vi "partial derivative.vi"(1 "x":dbl format="%0.2f", 2 "Coefficients":dbl[](array[numeric]) format="%0.2f") -> (0 "Partial Derivative":dbl[](array[numeric]) format="%0.5f")   [LabVIEW 2017, in "NI_AALPro.lvlib"]
uses:
  NI_AALPro.lvlib
panel:
  # "Partial Derivative"
  # "This VI takes an input x along with a number of coefficients to use in the Target Func NonLin vi and does a numerical computation of the partial derivative of the function with repect to each coefficient at value x."
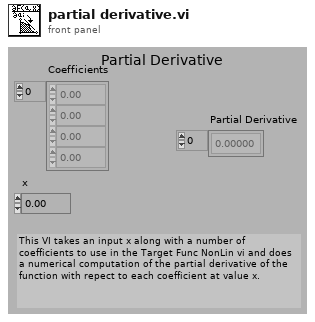
[diagram p1: front panel]
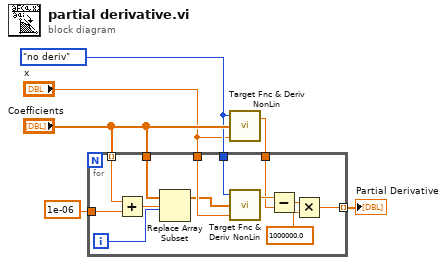
[diagram p0: block diagram]
diagram:
  w4 = enum16{"no deriv", "deriv"}."no deriv"
  n1 = call "Target Fnc & Deriv NonLin.vi"("X"="x", "Coefficients"="Coefficients", "Flag"=w4) -> ("Y"=w2:dbl)  [unwired: 1 out]
  n2 = for {
    tunnel: "x" -> [w13]
    tunnel: [w17] -> w6 mode=indexing
    tunnel: "Coefficients" -> [w12] mode=indexing
    tunnel: "Coefficients" -> [w16]
    tunnel: w4 -> [w9]
    tunnel: w2 -> [w8]
    tunnel: 1e-06 -> [w7]
    i -> [w14]
    n3 = Add(x=w12, y=w7) -> (x+y=w15:dbl)
    n4 = Replace Array Subset(array=w16, new element=w15, index=w14) -> (w10:dbl[])
    n5 = call "Target Fnc & Deriv NonLin.vi"("X"=w13, "Coefficients"=w10, "Flag"=w9) -> ("Y"=w11:dbl)  [unwired: 1 out]
    n6 = Subtract(x=w11, y=w8) -> (x-y=w18:dbl)
    n7 = Multiply(x=w18, y=1000000.0) -> (x*y=w17:dbl)
  }
  "Partial Derivative" <- w6
